vi "read Gcode.vi"(8 "error in":errorcluster, 9 "Parse comment lines":bool, 11 "Gcode path (use dialog)":path) -> (0 "error out":errorcluster, 2 "Gcode Array":string[](array[string]), 3 "Gcode path out":path)   [LabVIEW 2020]
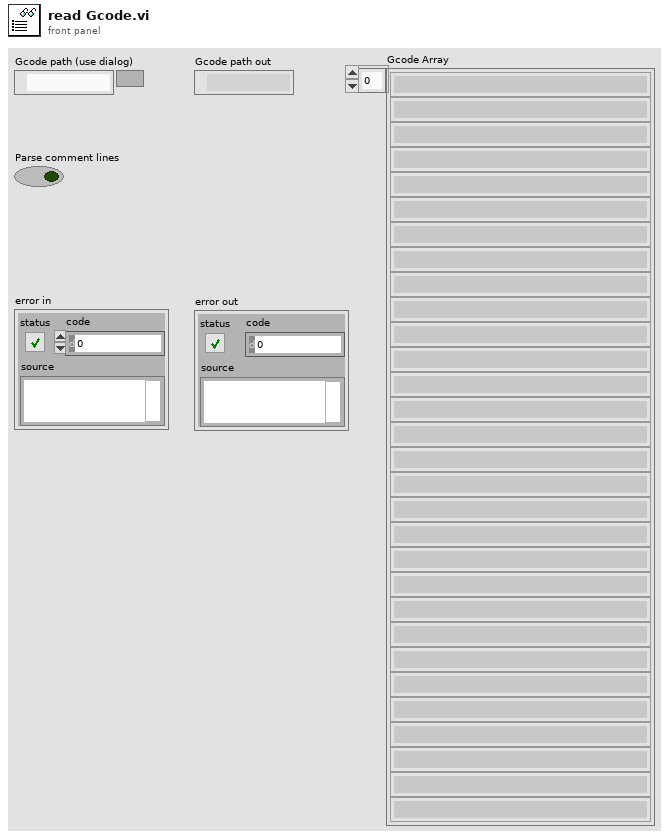
[diagram p1: front panel]
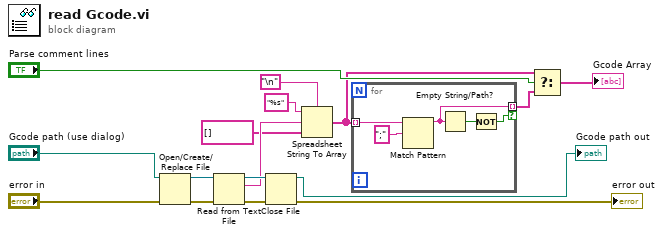
[diagram p0: block diagram]
diagram:
  n1 = Open/Create/Replace File(file path (use dialog)="Gcode path (use dialog)", error in="error in") -> (refnum out=w15:refnum<file>, error out=w14:errorcluster)  [unwired: 4 in, 1 out]
  n2 = Read from Text File(file (use dialog)=w15, error in=w14) -> (refnum out=w13:refnum<file>, text=w11:string, error out=w12:errorcluster)  [unwired: 2 in, 1 out]
  n3 = Close File(refnum=w13, error in=w12) -> (path=→"Gcode path out":path, error out=→"error out":errorcluster)
  n4 = Spreadsheet String To Array(delimiter (Tab)="\n", format string="%s", spreadsheet string=w11, array type (2D Dbl)=string[] []) -> (array=w1:string[])
  n5 = for {
    tunnel: w1 -> [w21] mode=indexing
    tunnel: [w19] -> w2 mode=indexing if=w17
    n6 = Match Pattern(string=w21, regular expression=";") -> (before substring=w19:string)  [unwired: 1 in, 3 out]
    n7 = Empty String/Path?(string/path=w19) -> (empty?=w18:bool)
    n8 = Not(x=w18) -> (.not. x?=w17:bool)
  }
  n9 = Select(t=w1, s="Parse comment lines", f=w2) -> (s? t:f=→"Gcode Array":string[])
